vi "CRYCalc Data item.vi"(0 "Data in":T1 {"Z data" items=["dB", "Lin"]; "X data" items=["dB", "Lin"]; "Y data" items=["dB", "Lin"]; "Z dB ref" format="%.1f"; "Z axis" items=["Log", "Lin"]; "X dB ref" format="%.1f"; "X axis" items=["Log", "Lin"]; "Y axis" items=["Log", "Lin"]; "Y dB ref" format="%.1f"; "Curve"."z" format="%.2f"; "Curve"."y" format="%.2f"; "Curve"."x" format="%.2f"}, 1 "Work in":u16, 2 "Mode xyz":u16, 3 "USL":dbl, 4 "LSL":dbl, 5 "Statistic Item":T3(ring), 6 "Step Setup VI No":i32, 7 "+/-Adjust(Deviation)":i32, 10 "Statistic Run Number":i32, 11 "rank number(best curve)":i32, 13 "rank number(worst curve)":i32) -> (14 "Data out":T1 {"Z data" items=["dB", "Lin"]; "X data" items=["dB", "Lin"]; "Y data" items=["dB", "Lin"]; "Z dB ref" format="%.1f"; "Z axis" items=["Log", "Lin"]; "X dB ref" format="%.1f"; "X axis" items=["Log", "Lin"]; "Y axis" items=["Log", "Lin"]; "Y dB ref" format="%.1f"; "Curve"."z" format="%.2f"; "Curve"."y" format="%.2f"; "Curve"."x" format="%.2f"})   [LabVIEW 2013]
uses:
  Typedef Control/CRYData Cluster Array.ctl
  Typedef Control/CRYData Cluster.ctl
  CRYStatistics Global.vi
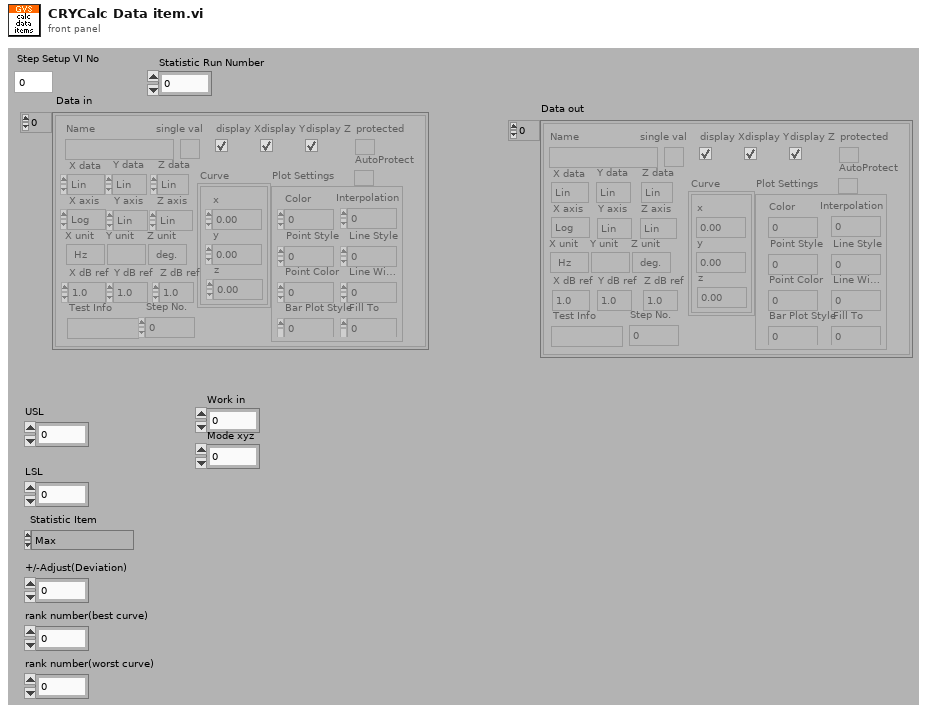
[diagram p1: front panel]
types:
  T1 = typedef "CRYData Cluster Array.ctl" = T2[]
  T2 = typedef "CRYData Cluster.ctl" = cluster{"Name":string, "Curve":cluster{"x":dbl, "y":dbl, "z":dbl}[], "X data":u16, "Y data":u16, "Z data":u16, "X axis":u16, "Y axis":u16, "Z axis":u16, "X unit":string, "Y unit":string, "Z unit":string, "X dB ref":dbl, "Y dB ref":dbl, "Z dB ref":dbl, "single val":bool, "protected":bool, "display X":bool, "display Y":bool, "display Z":bool, "Test Info":string, "Step No.":i32, "Plot Settings":cluster{"Color":u32, "Interpolation":u8, "Point Style":u8, "Line Style":u8, "Point Color":u32, "Line Width":u8, "Bar Plot Style":u8, "Fill To":i16}, "AutoProtect":bool}
  T3 = enum32{"Max", "Min", "Mean", "Absolute Standard Deviation", "Standard Deviation", "Pp", "Ppk", "Best Fit of Average", "Worst Fit of Average"}
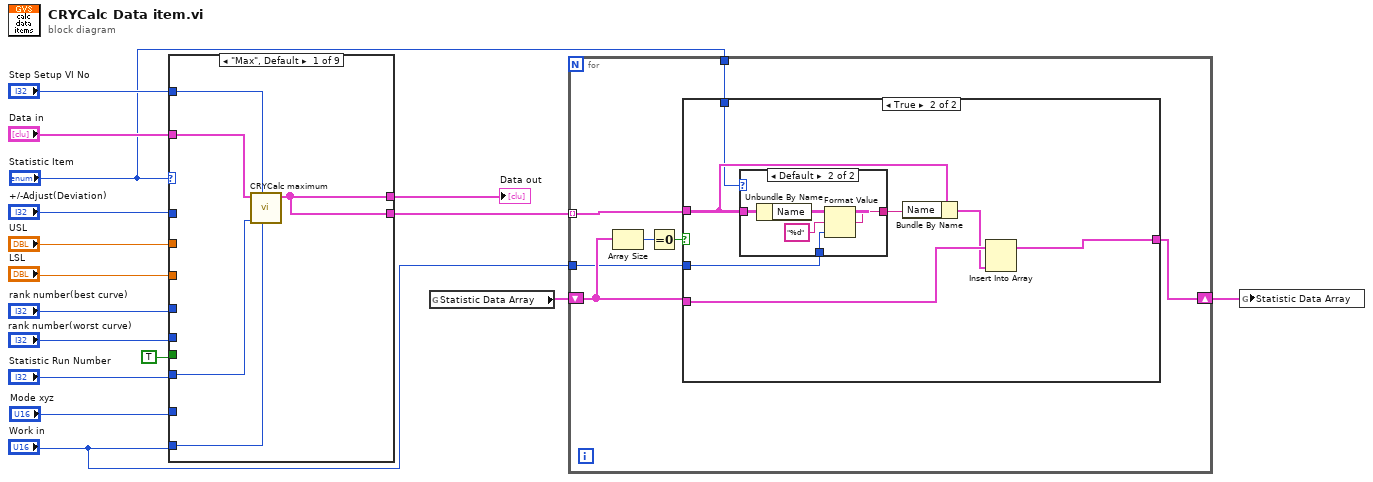
[diagram p0: block diagram]
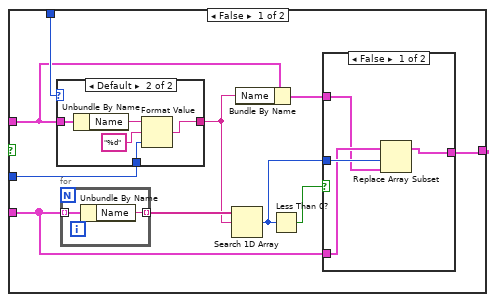
[diagram p2: hidden frame]
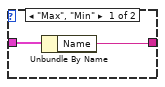
[diagram p3: hidden frame]
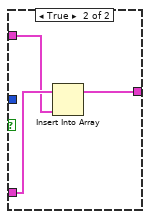
[diagram p4: hidden frame]
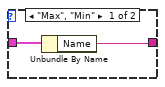
[diagram p5: hidden frame]
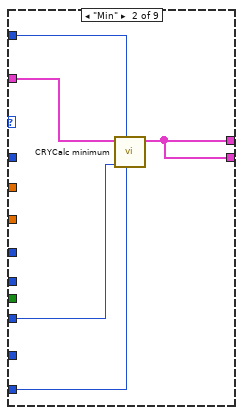
[diagram p6: hidden frame]
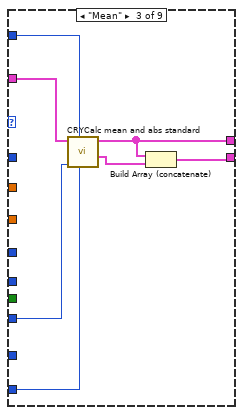
[diagram p7: hidden frame]
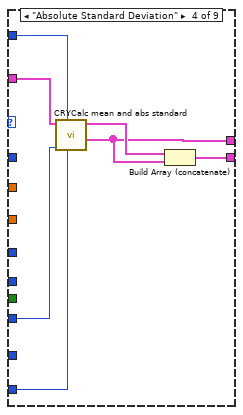
[diagram p8: hidden frame]
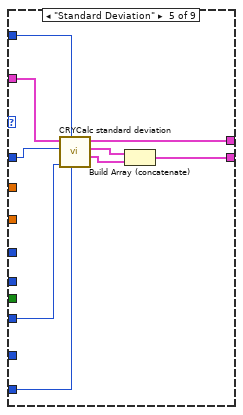
[diagram p9: hidden frame]
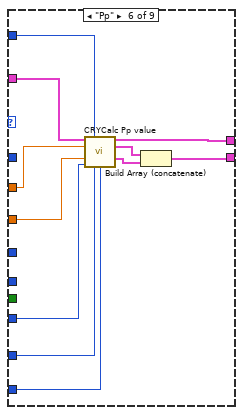
[diagram p10: hidden frame]
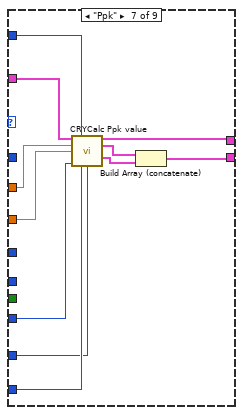
[diagram p11: hidden frame]
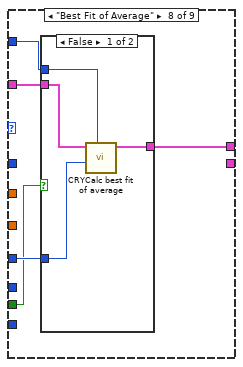
[diagram p12: hidden frame]
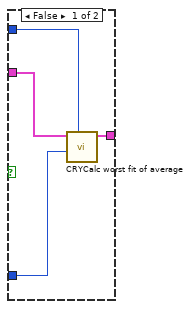
[diagram p15: hidden frame]
diagram:
  n1 = case shown="\"Max\", Default" "Statistic Item" {
    tunnel: "+/-Adjust(Deviation)" -> [_ _ _ _ w44 _ _ _ _]
    tunnel: "rank number(best curve)" -> [_ _ _ _ _ _ _ w74 _]
    tunnel: "rank number(worst curve)" -> [_ _ _ _ _ _ _ _ w83]
    tunnel: "USL" -> [_ _ _ _ _ w58 w69 _ _]
    tunnel: "LSL" -> [_ _ _ _ _ w57 w68 _ _]
    tunnel: "Data in" -> [w21 w26 w33 w37 w49 w59 w70 w75 w84]
    tunnel: [w20 w25 w32 w38 w48 w60 w71 w76 w85] -> w6
    tunnel: TRUE -> [_ _ _ _ _ _ _ w73 w82]
    tunnel: [w20 w25 w30 w39 w45 w54 w65 _ _] -> w8
    tunnel: "Step Setup VI No" -> [w19 w24 w29 w36 w43 w53 w64 w72 w81]
    tunnel: "Statistic Run Number" -> [w18 w23 w28 w35 w42 w51 w62 _ _]
    tunnel: "Work in" -> [w17 w22 w27 w34 w41 w52 w63 _ _]
    tunnel: "Mode xyz" -> [_ _ _ _ _ w50 w61 _ _]
    frame "Max", Default {
      n2 = call "CRYCalc maximum.vi"("Work in"=w17, "Step Setup VI No"=w19, "Statistic Run Number"=w18, "Data in"=w21) -> ("Maximum Out"=w20:T1)  [unwired: 2 in, 5 out]
    }
    frame "Min" {
      n3 = call "CRYCalc minimum.vi"("Work in"=w22, "Step Setup VI No"=w24, "Statistic Run Number"=w23, "Data in"=w26) -> ("Minimum Out"=w25:T1)  [unwired: 2 in, 5 out]
    }
    frame "Mean" {
      n4 = call "CRYCalc mean and abs standard.vi"("Work in"=w27, "Step Setup VI No"=w29, "Statistic Run Number"=w28, "Data in"=w33) -> ("Absolute StanDev Out"=w31:T1, "Mean Out"=w32:T1)  [unwired: 2 in, 4 out]
      n5 = Build Array (concatenate)(w32, w31) -> (w30:T1)
    }
    frame "Absolute Standard Deviation" {
      n6 = call "CRYCalc mean and abs standard.vi"("Work in"=w34, "Step Setup VI No"=w36, "Statistic Run Number"=w35, "Data in"=w37) -> ("Absolute StanDev Out"=w38:T1, "Mean Out"=w40:T1)  [unwired: 5 in, 1 out]
      n7 = Build Array (concatenate)(w40, w38) -> (w39:T1)
    }
    frame "Standard Deviation" {
      n8 = call "CRYCalc standard deviation.vi"("Work in"=w41, "Step Setup VI No"=w43, "Statistic Run Number"=w42, "+/-Adjust(Deviation)"=w44, "Data in"=w49) -> ("Absolute StanDev Out"=w46:T1, "Mean Out"=w47:T1, "Standard dev Out"=w48:T1)  [unwired: 1 in, 3 out]
      n9 = Build Array (concatenate)(w47, w46) -> (w45:T1)
    }
    frame "Pp" {
      n10 = call "CRYCalc Pp value.vi"("Data values in"=w59, "Step Setup VI No"=w53, "USL"=w58, "LSL"=w57, "Statistic Run Number"=w51, "Mode xyz"=w50, "Work in"=w52) -> ("Pp value Out"=w60:T1, "Mean Out"=w56:T1, "Absolute StanDev Out"=w55:T1)  [unwired: 6 in]
      n11 = Build Array (concatenate)(w56, w55) -> (w54:T1)
    }
    frame "Ppk" {
      n12 = call "CRYCalc Ppk value.vi"("Data values in"=w70, "Step Setup VI No"=w64, "USL"=w69, "LSL"=w68, "Statistic Run Number"=w62, "Work in"=w63, "Mode xyz"=w61) -> ("Ppk value Out"=w71:T1, "Mean Out"=w66:T1, "Absolute StanDev Out"=w67:T1)  [unwired: 6 in]
      n13 = Build Array (concatenate)(w66, w67) -> (w65:T1)
    }
    frame "Best Fit of Average" {
      n14 = case shown="False" w73 {
        tunnel: [w80 _] -> w76
        tunnel: w75 -> [w79 _]
        tunnel: w74 -> [w78 _]
        tunnel: w72 -> [w77 _]
        frame False {
          n15 = call "CRYCalc best fit of average.vi"("Step Setup VI No"=w77, "rank number(best curve)"=w78, "Data in"=w79) -> ("Best Fit Out"=w80:T1)  [unwired: 2 in, 6 out]
        }
        frame True {
        }
      }
    }
    frame "Worst Fit of Average" {
      n16 = case shown="True" w82 {
        tunnel: [w89 _] -> w85
        tunnel: w84 -> [w88 _]
        tunnel: w83 -> [w87 _]
        tunnel: w81 -> [w86 _]
        frame False {
          n17 = call "CRYCalc worst fit of average.vi"("Step Setup VI No"=w86, "rank number(worst curve)"=w87, "Data in"=w88) -> ("Worst Fit Out"=w89:T1)  [unwired: 1 in, 7 out]
        }
        frame True {
        }
      }
    }
  }
  "Data out" <- w6
  n18 = global read "CRYStatistics Global.vi" "Statistic Data Array"() -> (w10:T1)
  n19 = for {
    tunnel: w8 -> [w92] mode=indexing
    shift-right: [w94] -> w9
    shift-left: w10 -> [w93]
    tunnel: "Statistic Item" -> [w91]
    tunnel: "Work in" -> [w90]
    n20 = Array Size(array=w93) -> (size(s)=w96:i32)
    n21 = Equal To 0?(x=w96) -> (x = 0?=w95:bool)
    n22 = case shown="True" w95 {
      tunnel: [w103 w129] -> w94
      tunnel: w93 -> [w104 w128]
      tunnel: w92 -> [w99 w126]
      tunnel: w91 -> [w101 w124]
      tunnel: w90 -> [w100 w123]
      frame False {
        n23 = case shown="Default" w101 {
          tunnel: [w107 w109] -> w98
          tunnel: w99 -> [w108 w113]
          tunnel: w100 -> [_ w110]
          frame "Max", "Min" {
            n24 = Unbundle By Name(w108) -> ("Name"=w107:string)
          }
          frame Default {
            n25 = Unbundle By Name(w113) -> ("Name"=w111:string)
            n26 = Format Value(string ("")=w111, format string="%d", value (0)=w110) -> (output string=w109:string)
          }
        }
        n27 = for {
          tunnel: w104 -> [w122] mode=indexing
          tunnel: [w121] -> w106 mode=indexing
          n28 = Unbundle By Name(w122) -> ("Name"=w121:string)
        }
        n29 = Search 1D Array(1D array=w106, element=w98) -> (index of element=w102:i32)  [unwired: 1 in]
        n30 = Bundle By Name(cluster=w99, "Name"=w98) -> (w97:T2)
        n31 = Less Than 0?(x=w102) -> (x < 0?=w105:bool)
        n32 = case shown="False" w105 {
          tunnel: w104 -> [w116 w120]
          tunnel: w97 -> [w115 w119]
          tunnel: [w114 w118] -> w103
          tunnel: w102 -> [w117 _]
          frame False {
            n33 = Replace Array Subset(array=w116, new element=w115, index=w117) -> (w114:T1)
          }
          frame True {
            n34 = Insert Into Array(array=w120, new element=w119) -> (w118:T1)  [unwired: 1 in]
          }
        }
      }
      frame True {
        n35 = case shown="Default" w124 {
          tunnel: [w130 w132] -> w127
          tunnel: w126 -> [w131 w136]
          tunnel: w123 -> [_ w133]
          frame "Max", "Min" {
            n36 = Unbundle By Name(w131) -> ("Name"=w130:string)
          }
          frame Default {
            n37 = Unbundle By Name(w136) -> ("Name"=w134:string)
            n38 = Format Value(string ("")=w134, format string="%d", value (0)=w133) -> (output string=w132:string)
          }
        }
        n39 = Bundle By Name(cluster=w126, "Name"=w127) -> (w125:T2)
        n40 = Insert Into Array(array=w128, new element=w125) -> (w129:T1)  [unwired: 1 in]
      }
    }
  }
  n41 = global write "CRYStatistics Global.vi" "Statistic Data Array"(w9) -> ()
